vi "Automatic Tap.vi"() -> ()   [LabVIEW 2022 SP3]
uses:
  TapStateMachineControl.ctl
panel:
  out "millisecond timer value 2":u32
  out "millisecond timer value":u32
  out "Hand in Time":u32
  in  "Hands Inserted":bool
  in  "?":bool
  out "Hand Out Time":u32
  in  "Time Untiil Tap Off":u32
  in  "Time Until Tap On":u32
  out "Tap on":bool
  out "State":T1
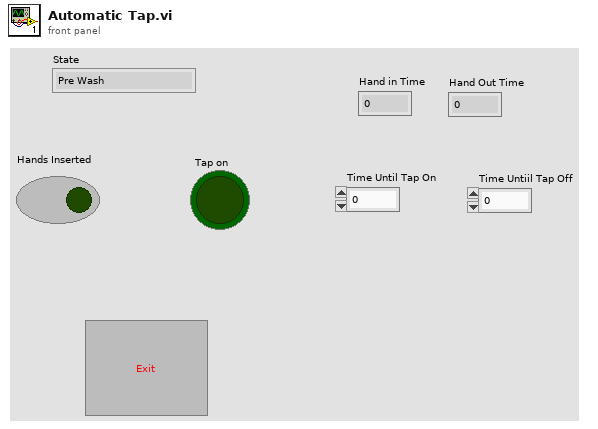
[diagram p1: front panel]
types:
  T1 = typedef "TapStateMachineControl.ctl" = enum16{"Pre Wash", "Check Timer1", "Tap On", "Check Timer 2"}
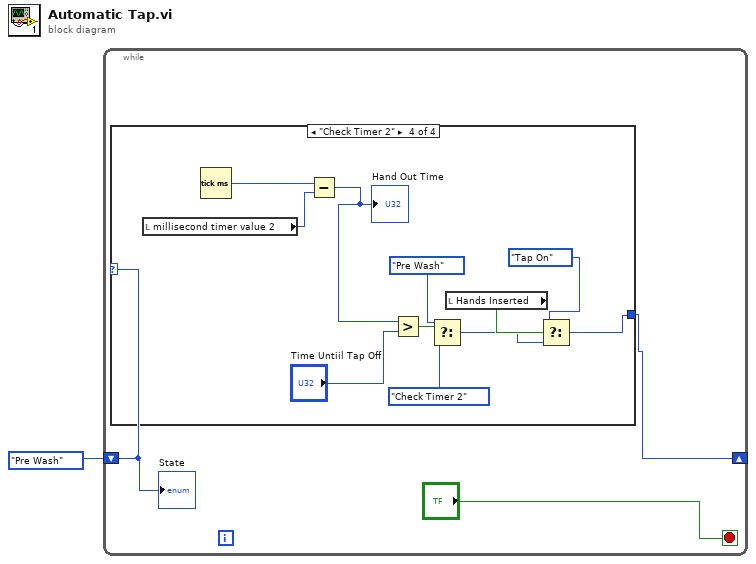
[diagram p0: block diagram]
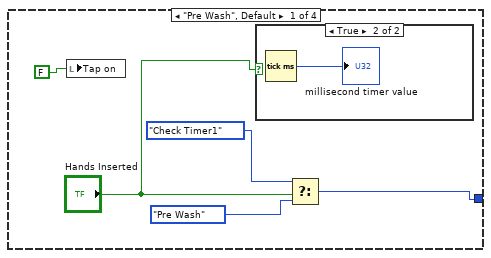
[diagram p2: hidden frame]
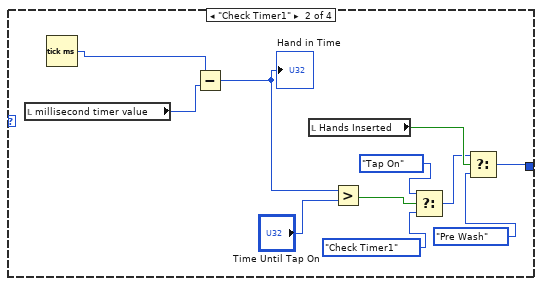
[diagram p4: hidden frame]
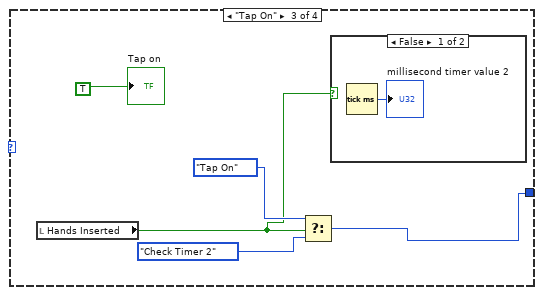
[diagram p5: hidden frame]
diagram:
  n1 = while {
    shift-right: [w4] -> _
    shift-left: TapStateMachineControl."Pre Wash" ("State") -> [w3]
    stop <- "?" stop-if-true
    n2 = case shown="\"Check Timer 2\"" w3 {
      tunnel: [w5 w11 w22 w28] -> w4
      frame "Pre Wash", Default {
        n3 = local write "Tap on"(FALSE) -> ()
        n4 = case shown="True" "Hands Inserted" {
          frame False {
          }
          frame True {
            n5 = Tick Count (ms)() -> (millisecond timer value=→"millisecond timer value":u32)
          }
        }
        n6 = Select(t=TapStateMachineControl."Check Timer1" ("State"), s="Hands Inserted", f=TapStateMachineControl."Pre Wash" ("State")) -> (s? t:f=w5:T1)
      }
      frame "Check Timer1" {
        n7 = local read "millisecond timer value"() -> (w20:u32)
        n8 = Tick Count (ms)() -> (millisecond timer value=w21:u32)
        n9 = Subtract(x=w21, y=w20) -> (x-y=w19:u32)
        "Hand in Time" <- w19
        n10 = local read "Hands Inserted"() -> (w14:bool)
        n11 = Greater?(x=w19, y="Time Until Tap On") -> (0:w17:bool)
        n12 = Select(t=TapStateMachineControl."Tap On" ("State"), s=w17, f=TapStateMachineControl."Check Timer1" ("State")) -> (s? t:f=w13:T1)
        n13 = Select(t=w13, s=w14, f=TapStateMachineControl."Pre Wash" ("State")) -> (s? t:f=w11:T1)
      }
      frame "Tap On" {
        n14 = local read "Hands Inserted"() -> (w23:bool)
        n15 = Select(t=TapStateMachineControl."Tap On" ("State"), s=w23, f=TapStateMachineControl."Check Timer 2" ("State")) -> (s? t:f=w22:T1)
        n16 = case shown="False" w23 {
          frame False {
            n17 = Tick Count (ms)() -> (millisecond timer value=→"millisecond timer value 2":u32)
          }
          frame True {
          }
        }
        "Tap on" <- TRUE
      }
      frame "Check Timer 2" {
        n18 = local read "millisecond timer value 2"() -> (w37:u32)
        n19 = Tick Count (ms)() -> (millisecond timer value=w38:u32)
        n20 = Subtract(x=w38, y=w37) -> (x-y=w36:u32)
        "Hand Out Time" <- w36
        n21 = Greater?(x=w36, y="Time Untiil Tap Off") -> (0:w34:bool)
        n22 = Select(t=TapStateMachineControl."Pre Wash" ("State"), s=w34, f=TapStateMachineControl."Check Timer 2" ("State")) -> (s? t:f=w30:T1)
        n23 = local read "Hands Inserted"() -> (w31:bool)
        n24 = Select(t=TapStateMachineControl."Tap On" ("State"), s=w31, f=w30) -> (s? t:f=w28:T1)
      }
    }
    "State" <- w3
  }
